vi "get MAC address.vi"() -> (3 "MAC address":string)   [LabVIEW 2024, in "LabView SystemInfo Library.lvlib"]
uses:
  LabView SystemInfo Library.lvlib
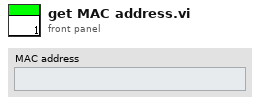
[diagram p1: front panel]
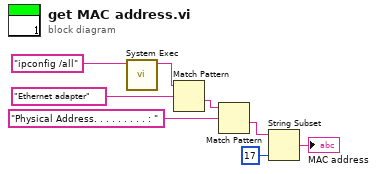
[diagram p0: block diagram]
diagram:
  n1 = call <vilib>:"System Exec.vi"("command line"="ipconfig /all") -> ("standard output"=w7:string)  [unwired: 7 in, 3 out]
  n2 = Match Pattern(string=w7, regular expression="Ethernet adapter") -> (after substring=w5:string)  [unwired: 1 in, 3 out]
  n3 = Match Pattern(string=w5, regular expression="Physical Address. . . . . . . . . : ") -> (after substring=w3:string)  [unwired: 1 in, 3 out]
  n4 = String Subset(string=w3, length (rest)=17 ("length (rest)")) -> (substring=→"MAC address":string)  [unwired: 1 in]
